vi "Modules - Manual Control.vi"() -> ()   [LabVIEW 2019]
uses:
  Controls/Manual - State.ctl
  Controls/eFGV States.ctl
  Controls/Manual - Data Structure.ctl
  Controls/UDP - Command.ctl
  Controls/Communication - Write Data.ctl
  Controls/Global - IP Address.vi
  Controls/Global - Device.vi
  Controls/Global - Test.vi
  Controls/Global - Channel.vi
  Controls/Global - Unit.vi
  Controls/Global - System.vi
panel:
  in  "Device Name":string
  in  "Zero Ch4":bool
  in  "Zero Ch3":bool
  out "Slide":u8(slide) scale=0.0..1.0
  out "Label Ch4":string caption="Cell Pressure Transducer"
  out "Data Ch4":sgl format="%.2f"
  out "Label Ch3":string caption="Cell Pressure Transducer"
  out "Data Ch3":sgl format="%.2f"
  out "Status":u16(ring) caption="Event" items=["Stop", "Ramp Up", "Ramp Down", "Jog Up", "Jog Down", "PID Mode", "PID Ramp"]
  out "Event":u16(ring) caption="Status" items=["Stop", "Running", "PID", "Up Limit", "Down Limit", "Load Limit"]
  out "Unit Ch2b":string caption="Cell Pressure Transducer"
  in  "Speed":sgl format="%.3f"
  out "Unit Ch2":string caption="Cell Pressure Transducer"
  in  "Setpoint Ch2":sgl
  in  "Target 2":bool
  out "Label Ch1":string caption="Cell Pressure Transducer"
  out "Unit Ch1b":string caption="Cell Pressure Transducer"
  out "Unit Ch1":string caption="Cell Pressure Transducer"
  out "Data Ch2":sgl format="%.3f"
  out "Data Ch1":sgl caption="Load" format="%.3f"
  in  "Setpoint Rate":sgl format="%.3f"
  in  "Stop Ch2":bool
  in  "Ramp":bool
  in  "Zero Ch2":bool
  in  "Setpoint Ch1":sgl
  in  "Stop Ch1":bool
  in  "Target":bool
  in  "Zero Ch1":bool
  in  "Select Machine":u16(ring) items=["Please Select", "TEST"]
  in  "MStop":bool
  in  "Fast down":bool
  in  "Down":bool
  in  "Fast Up":bool
  in  "Up":bool
  out "Label Ch2":string caption="Cell Pressure Transducer"
  # "(         /min)"
  # "/min"
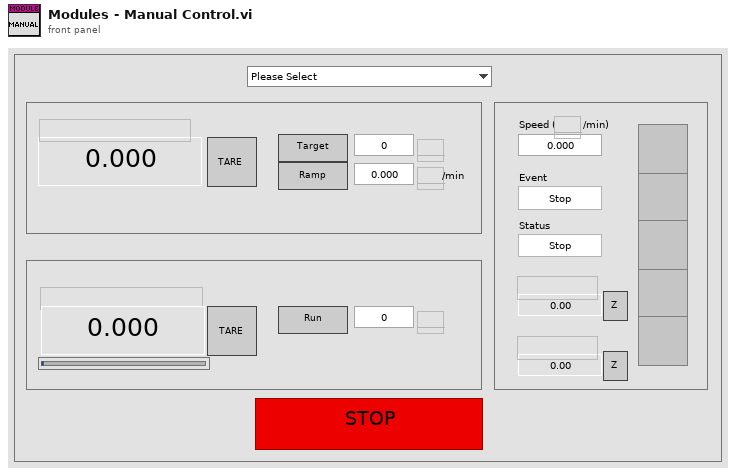
[diagram p1: front panel]
types:
  T1 = enum8{"Enabled", "Disabled", "Disabled and Grayed Out"}
  T2 = typedef "Manual - State.ctl" = enum16{"Init", "Idle", "Read Data", "Stop", "Panel Close", "Close", "Exit"}
  T3 = cluster{"Up":bool, "FUp":bool, "Dn":bool, "FDn":bool, "Running?":bool}
  T4 = typedef "Manual - Data Structure.ctl" = cluster{"Dir":bool, "Device Running?":bool[], "Selected":u16, "PID":cluster{"Output Range":cluster{"High":dbl, "Low":dbl}, "PID Tuning":cluster{"(Kc)":dbl, " (Ti, min)":dbl, "(Td, min)":dbl}, "SetPoint":dbl}, "Machine Table":string[][], "PID Type":enum32{"Sensor", "Displacement"}, "Ramp duration":i32, "i Ramp":i32, "R Elapse":dbl, "R Done":bool, "R To":dbl, "Ramp":bool, "Device Name":string[], "Inv":cluster{"M":i32[], "Bool":bool[]}, "MRun?":bool, "M":cluster{"Up":bool, "FUp":bool, "Dn":bool, "FDn":bool, "Running?":bool}[], "P Target":dbl, "Device IP":string[], "Selected Device":string}
  T5 = enum16{"New Test", "Test Plan", "Job Record", "Instrument", "Machine", "Station", "Machine Control"}
  T6 = typedef "UDP - Command.ctl" = enum16{"Stop", "Jog Up", "Jog Down", "Ramp Up", "Ramp Down", "PID Target", "PID Ramp", "Disp Run", "Read Ch Data", "Zero Channel", "Zero Disp", "Read Sensor", "Write Sensor", "Read ADC", "Write ADC", "Read PID", "Write PID", "Read Test", "Write Test", "Read System", "Write System", "Read Datalog", "Read Datalog Sensor"}
  T7 = typedef "Communication - Write Data.ctl" = cluster{"Test":cluster{"Target Load":sgl, "Target Disp":sgl, "Rate":sgl, "Speed":sgl}, "Sensor":cluster{"Name":string[], "Unit":string[], "Decimal Point":u8[], "Ch Log":u8[], "H Alarm":u8[], "L Alarm":u8[], "H Limit":sgl[], "L Limit":sgl[], "Filter":u8[], "Gain":u8[], "Calib Type":u32[]}, "PID":cluster{"SP":sgl, "PV":sgl, "kP":sgl, "kI":sgl, "kD":sgl, "FF":sgl, "Err Band":sgl, "Max":i32, "Min":i32, "Ts":u32, "Out":i32, "Mode":u8}, "ADC":cluster{"Active Ch":u8[], "Filter Type":u8, "Post Filter":u8[], "Gain":u8[], "FS":u16, "IntOC":u8, "IntFC":u8, "SysOC":u8, "Cofficient":dbl[], "K":dbl[], "Max":i32}, "System":cluster{"Out Type":u8, "Inverse":u8, "Monitor":u8, "Reserve":u8, "ACC Time":u32, "Pulse Rev":u32, "Stroke":u32, "Auto Off":u32, "Gear Ratio":sgl, "Pitch":sgl, "Max Speed":u32, "Jog Speed":u32, "Disp Coff":sgl, "Max Load":u32}, "Index":enum16{"Ch1", "Ch2", "Ch3", "Ch4", "Ch5", "Ch6", "Ch7", "Ch8", "Ch9", "Ch10", "Ch11", "Ch12", "Ch13", "Ch14", "Ch15", "Ch16"}, "Datalog":enum16{"Ch1-Ch16", "Ch17-Ch32", "Ch32-Ch48", "Ch49-Ch64", "Empty"}}
  T8 = enum16{"Ch1", "Ch2", "Ch3", "Ch4", "Ch5", "Ch6", "Ch7", "Ch8", "Ch9", "Ch10", "Ch11", "Ch12", "Ch13", "Ch14", "Ch15", "Ch16"}
  T9 = typedef "eFGV States.ctl" = enum16{"Init", "Read", "Write", "Exit"}
  T10 = cluster{"Up":bool, "FUp":bool, "Dn":bool, "FDn":bool, "Running?":bool}[]
  T11 = cluster{"Target Load":sgl, "Target Disp":sgl, "Rate":sgl, "Speed":sgl}[]
  T12 = cluster{"Target Load":sgl, "Target Disp":sgl, "Rate":sgl, "Speed":sgl}
  T13 = cluster{"Out Type":u8, "Inverse":u8, "Monitor":u8, "Reserve":u8, "ACC Time":u32, "Pulse Rev":u32, "Stroke":u32, "Auto Off":u32, "Gear Ratio":sgl, "Pitch":sgl, "Max Speed":u32, "Jog Speed":u32, "Disp Coff":sgl, "Max Load":u32}[]
  T14 = typedef "UDP - Event.ctl" = u16
  T15 = typedef "UDP - Status.ctl" = u16
  T16 = cluster{"Channels":cluster{"Ch1":sgl, "Ch2":sgl, "Ch3":sgl, "Ch4":sgl, "Ch5":sgl, "Ch6":sgl, "Ch7":sgl, "Ch8":sgl, "Ch9":sgl, "Ch10":sgl, "Ch11":sgl, "Ch12":sgl, "Ch13":sgl, "Ch14":sgl, "Ch15":sgl, "Ch16":sgl}, "Event":T14, "Status":T15, "IP":string}[]
  T17 = cluster{"Channels":cluster{"Ch1":sgl, "Ch2":sgl, "Ch3":sgl, "Ch4":sgl, "Ch5":sgl, "Ch6":sgl, "Ch7":sgl, "Ch8":sgl, "Ch9":sgl, "Ch10":sgl, "Ch11":sgl, "Ch12":sgl, "Ch13":sgl, "Ch14":sgl, "Ch15":sgl, "Ch16":sgl}, "Event":T14, "Status":T15, "IP":string}
  T18 = cluster{"Out Type":u8, "Inverse":u8, "Monitor":u8, "Reserve":u8, "ACC Time":u32, "Pulse Rev":u32, "Stroke":u32, "Auto Off":u32, "Gear Ratio":sgl, "Pitch":sgl, "Max Speed":u32, "Jog Speed":u32, "Disp Coff":sgl, "Max Load":u32}
  T19 = cluster{"Name":string[], "Unit":string[], "Decimal Point":u8[], "Ch Log":u8[], "H Alarm":u8[], "L Alarm":u8[], "H Limit":sgl[], "L Limit":sgl[], "Filter":u8[], "Gain":u8[], "Calib Type":u32[]}[]
  T20 = cluster{"Name":string[], "Unit":string[], "Decimal Point":u8[], "Ch Log":u8[], "H Alarm":u8[], "L Alarm":u8[], "H Limit":sgl[], "L Limit":sgl[], "Filter":u8[], "Gain":u8[], "Calib Type":u32[]}
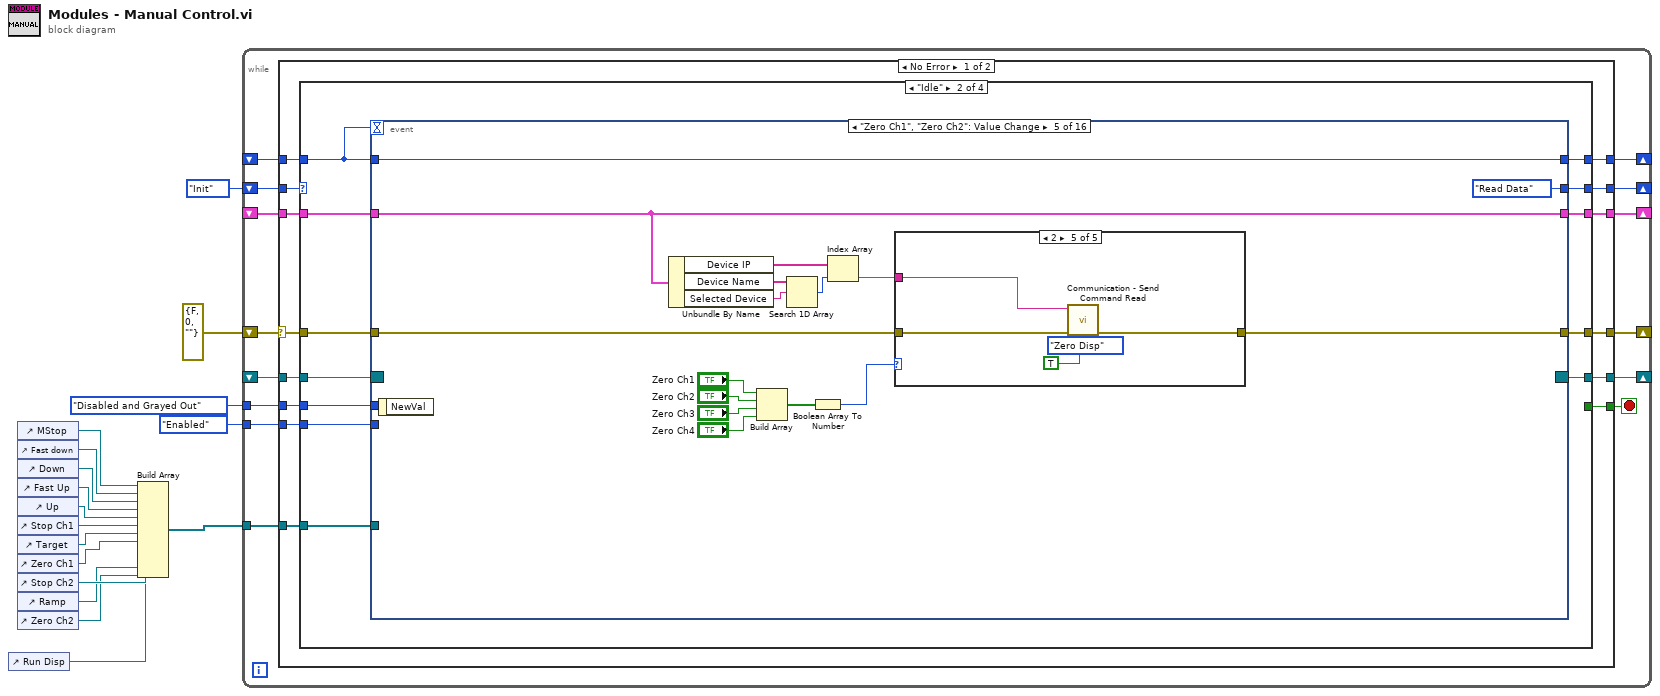
[diagram p0: block diagram]
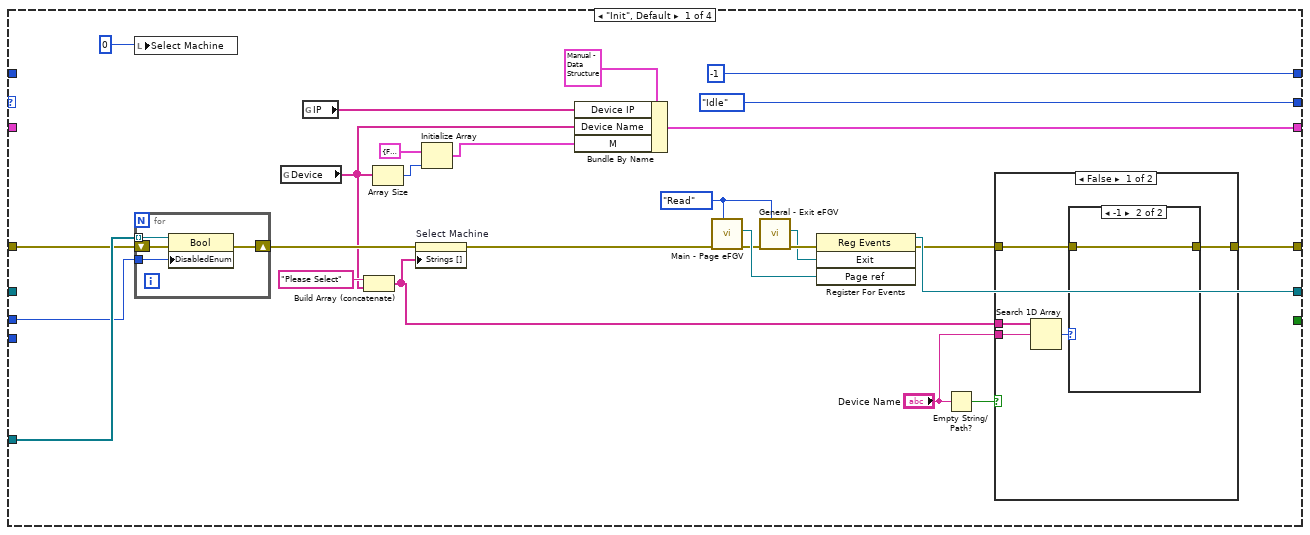
[diagram p2: hidden frame]
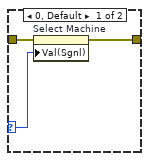
[diagram p3: hidden frame]
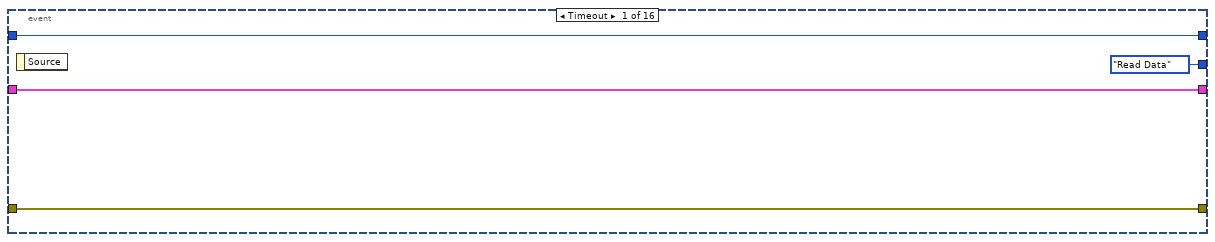
[diagram p5: hidden frame]
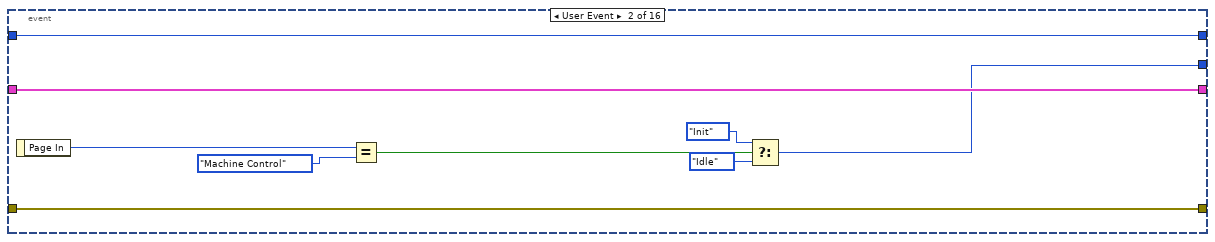
[diagram p6: hidden frame]
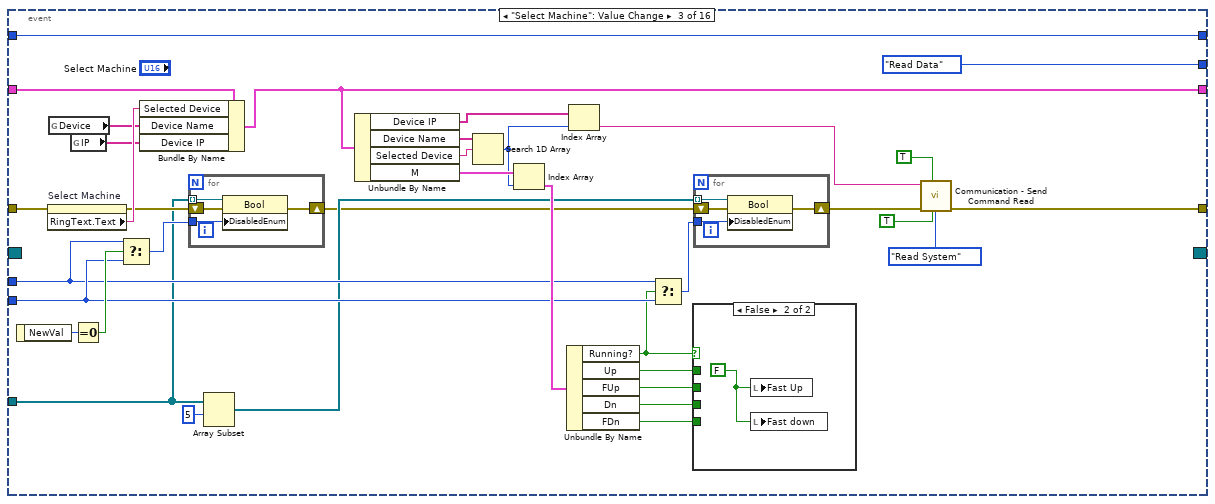
[diagram p7: hidden frame]
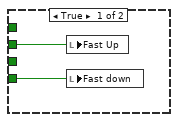
[diagram p8: hidden frame]
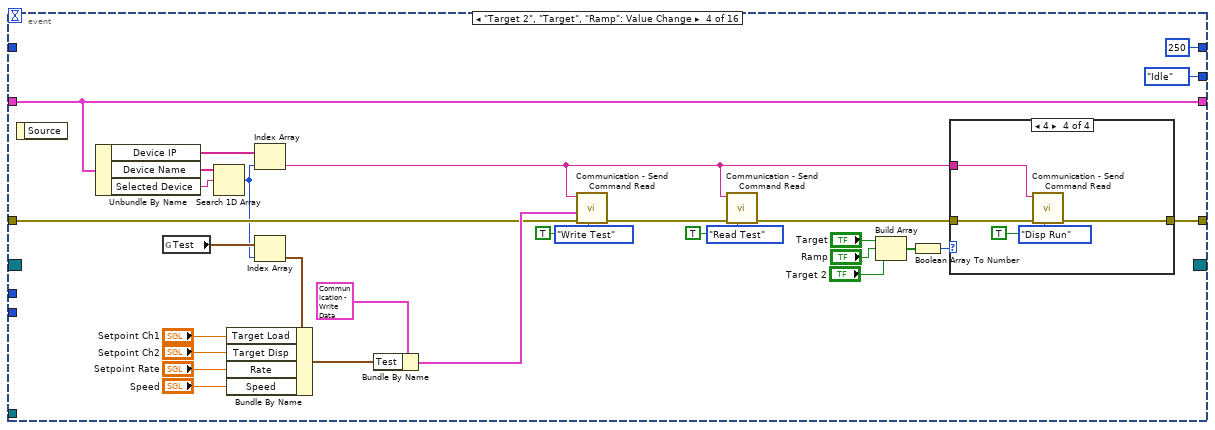
[diagram p9: hidden frame]
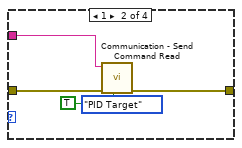
[diagram p11: hidden frame]
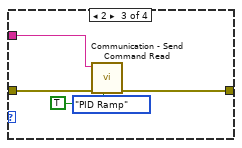
[diagram p12: hidden frame]
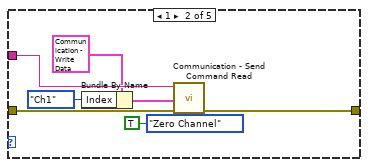
[diagram p14: hidden frame]
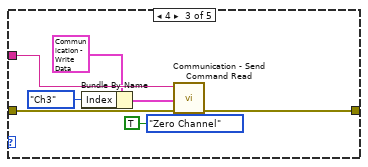
[diagram p15: hidden frame]
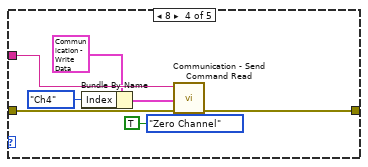
[diagram p16: hidden frame]
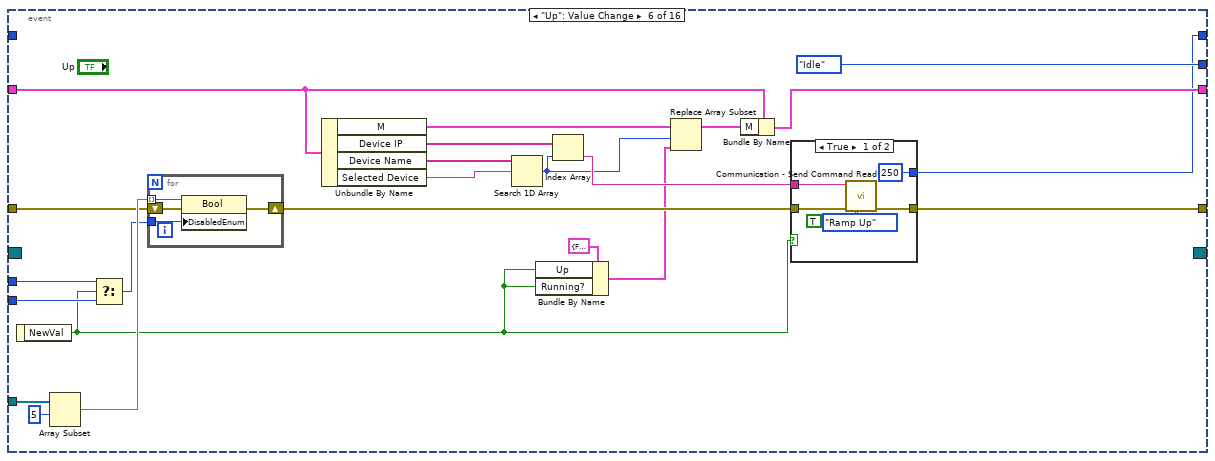
[diagram p17: hidden frame]
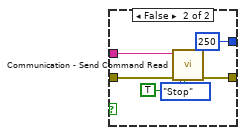
[diagram p18: hidden frame]
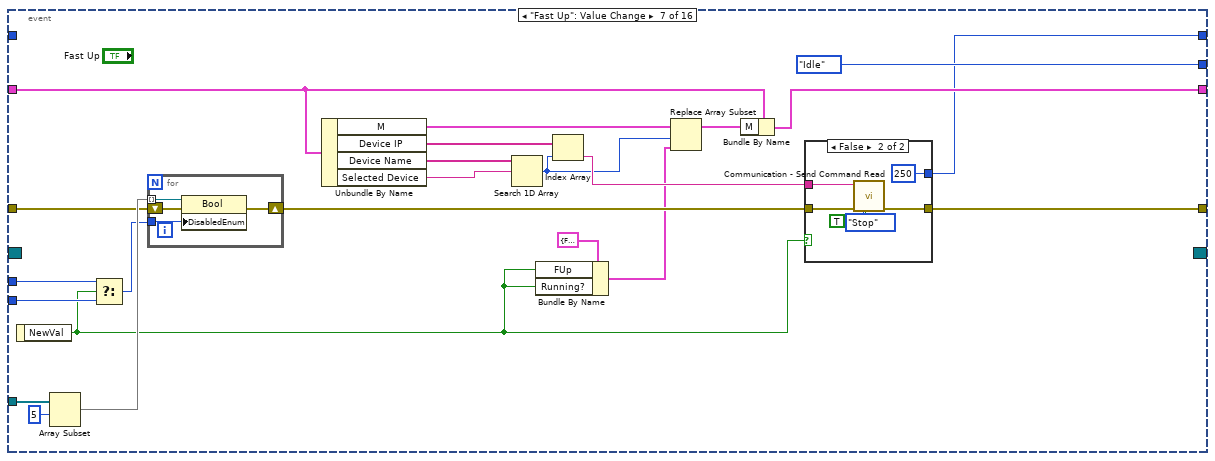
[diagram p19: hidden frame]
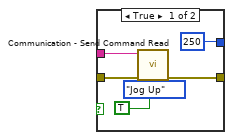
[diagram p20: hidden frame]
diagram:
  n1 = control-ref of="Run Disp"() -> (w1:refnum<vi>)
  n2 = control-ref of="MStop"() -> (w15:refnum<vi>)
  n3 = control-ref of="Fast down"() -> (w14:refnum<vi>)
  n4 = control-ref of="Down"() -> (w13:refnum<vi>)
  n5 = control-ref of="Fast Up"() -> (w12:refnum<vi>)
  n6 = control-ref of="Up"() -> (w11:refnum<vi>)
  n7 = control-ref of="Stop Ch1"() -> (w10:refnum<vi>)
  n8 = control-ref of="Target"() -> (w9:refnum<vi>)
  n9 = control-ref of="Zero Ch1"() -> (w8:refnum<vi>)
  n10 = control-ref of="Stop Ch2"() -> (w7:refnum<vi>)
  n11 = control-ref of="Ramp"() -> (w6:refnum<vi>)
  n12 = control-ref of="Zero Ch2"() -> (w5:refnum<vi>)
  n13 = Build Array(w15, w14, w13, w12, w11, w10, w9, w8, w7, w6, w5, w1) -> (w4:refnum<vi>[])
  n14 = while {
    shift-right: [w29] -> _
    shift-left: errorcluster {"status"=FALSE, "code"=0, "source"=""} ("error constant") -> [w31]
    shift-right: [w28] -> _
    shift-left: Manual_-_State."Init" -> [w30]
    shift-right: [w26] -> _
    shift-left: _ -> [w25]
    shift-right: [w24] -> _
    shift-left: _ -> [w23]
    shift-right: [w22] -> _
    shift-left: _ -> [w21]
    tunnel: w4 -> [w20]
    tunnel: T1."Disabled and Grayed Out" ("Disabled") -> [w19]
    tunnel: T1."Enabled" ("Disabled") -> [w18]
    stop <- w27 stop-if-true
    n15 = case shown="No Error" w31 {
      selector: w31 -> [w43 w617]
      tunnel: w30 -> [w45 _]
      tunnel: [w44 w618] -> w29
      tunnel: [w42 Manual_-_State."Idle"] -> w28
      tunnel: [w41 _] -> w27
      tunnel: [w40 w625] -> w26
      tunnel: w25 -> [w39 w625]
      tunnel: [w38 w628] -> w24
      tunnel: w23 -> [w37 w628]
      tunnel: [w36 w627] -> w22
      tunnel: w21 -> [w35 w627]
      tunnel: w20 -> [w34 _]
      tunnel: w19 -> [w33 _]
      tunnel: w18 -> [w32 _]
      frame No Error {
        n16 = case shown="\"Idle\"" w45 {
          tunnel: [w49 w92 w577 w610] -> w44
          tunnel: w43 -> [w51 w91 w566 w609]
          tunnel: [Manual_-_State."Idle" w98 Manual_-_State."Idle" Manual_-_State."Close"] -> w42
          tunnel: [_ _ _ TRUE] -> w41
          tunnel: [-1 w97 w596 -1] -> w40
          tunnel: w39 -> [_ w87 w596 _]
          tunnel: [w68 w95 w595 w613] -> w38
          tunnel: w37 -> [_ w96 w595 w613]
          tunnel: [w57 w94 w593 T4 {"Dir"=FALSE, "Device Running?"=[], "Selected"=0, "PID"={"Output Range"={"High"=100.0, "Low"=-100.0}, "PID Tuning"={"(Kc)"=1.0, " (Ti, min)"=0.01, "(Td, min)"=0.0}, "SetPoint"=0.0}, "Machine Table"=[], "PID Type"=enum."Sensor", "Ramp duration"=0, "i Ramp"=0, "R Elapse"=0.0, "R Done"=FALSE, "R To"=0.0, "Ramp"=FALSE, "Device Name"=[], "Inv"={"M"=[], "Bool"=[]}, "MRun?"=FALSE, "M"=[], "P Target"=0.0, "Device IP"=[], "Selected Device"=""}] -> w36
          tunnel: w35 -> [_ w93 w593 _]
          tunnel: w34 -> [w64 w90 _ _]
          tunnel: w33 -> [w62 w89 _ _]
          tunnel: w32 -> [_ w88 _ _]
          frame "Init", Default {
            w65 = eFGV_States."Read" ("Action")
            n17 = local write "Select Machine"(0) -> ()
            n18 = for {
              shift-right: [w85] -> w60
              shift-left: w51 -> [w86]
              tunnel: w64 -> [w84] mode=indexing
              tunnel: w62 -> [w83]
              n19 = property class="Bool"(reference=w84, error in=w86, "DisabledEnum"=w83) -> (error out=w85:errorcluster)  [unwired: 1 out]
            }
            n20 = global read "Global - Device.vi" "Device"() -> (w53:string[])
            n21 = global read "Global - IP Address.vi" "IP"() -> (w52:string[])
            n22 = Build Array (concatenate)("Please Select", w53) -> (w47:string[])
            n23 = Array Size(array=w53) -> (size(s)=w56:i32)
            n24 = property on="Select Machine" class="Ring (strict)"(error in=w60, "Strings []"=w47) -> (error out=w59:errorcluster)  [unwired: 1 in, 1 out]
            n25 = Initialize Array(T3 {"Up"=FALSE, "FUp"=FALSE, "Dn"=FALSE, "FDn"=FALSE, "Running?"=FALSE} ("M"), w56) -> (w54:T10)
            n26 = Bundle By Name(cluster=T4 {"Dir"=FALSE, "Device Running?"=[], "Selected"=0, "PID"={"Output Range"={"High"=100.0, "Low"=-100.0}, "PID Tuning"={"(Kc)"=1.0, " (Ti, min)"=0.01, "(Td, min)"=0.0}, "SetPoint"=0.0}, "Machine Table"=[], "PID Type"=enum."Sensor", "Ramp duration"=0, "i Ramp"=0, "R Elapse"=0.0, "R Done"=FALSE, "R To"=0.0, "Ramp"=FALSE, "Device Name"=[], "Inv"={"M"=[], "Bool"=[]}, "MRun?"=FALSE, "M"=[], "P Target"=0.0, "Device IP"=[], "Selected Device"=""}, "Device IP"=w52, "Device Name"=w53, "M"=w54) -> (w57:T4)
            n27 = call "Main - Page eFGV.vi"("eFGV States"=w65, "error in (no error)"=w59) -> ("error out"=w63:errorcluster, "Page ref"=w66:refnum<user-event>)  [unwired: 7 in, 1 out]
            n28 = call "General - Exit eFGV.vi"("eFGV States"=w65, "error in (no error)"=w63) -> ("error out"=w70:errorcluster, "Exit"=w69:refnum<user-event>)  [unwired: 7 in, 1 out]
            n29 = register-events(error in=w70, w69, w66) -> (reference out=w68:refnum<event-registration>, error out=w48:errorcluster)  [unwired: 1 in]
            n30 = Empty String/Path?(string/path="Device Name") -> (empty?=w50:bool)
            n31 = case shown="False" w50 {
              tunnel: [w74 w82] -> w49
              tunnel: w48 -> [w75 w82]
              tunnel: w47 -> [w77 _]
              tunnel: "Device Name" -> [w76 _]
              frame False {
                n32 = Search 1D Array(1D array=w77, element=w76) -> (index of element=w73:i32)  [unwired: 1 in]
                n33 = case shown="-1" w73 {
                  selector: w73 -> [w78 _]
                  tunnel: w75 -> [w80 w81]
                  tunnel: [w79 w81] -> w74
                  frame 0, Default {
                    n34 = property on="Select Machine" class="Ring (strict)"(error in=w80, "Val(Sgnl)"=w78) -> (error out=w79:errorcluster)  [unwired: 1 in, 1 out]
                  }
                  frame -1 {
                  }
                }
              }
              frame True {
              }
            }
          }
          frame "Idle" {
            n35 = event shown="[4] \"Zero Ch1\", \"Zero Ch2\": Value Change" {
              selector: w96 -> [_ _ _ _ _ _ _ _ _ _ _ _ _ _ _ _]
              dyn-events: [_ _ _ _ _ _ _ _ _ _ _ _ _ _ _ _] -> w95
              timeout: w87 -> [_ _ _ _ _ _ _ _ _ _ _ _ _ _ _ _]
              tunnel: [w102 w111 w116 w183 w207 w252 w300 w339 w378 w423 w434 w455 w476 w497 w521 w537] -> w92
              tunnel: w91 -> [w102 w111 w144 w165 w211 w267 w306 w345 w384 w428 w450 w471 w492 w513 w520 w538]
              tunnel: [Manual_-_State."Read Data" w104 Manual_-_State."Read Data" Manual_-_State."Idle" Manual_-_State."Read Data" Manual_-_State."Idle" Manual_-_State."Idle" Manual_-_State."Idle" Manual_-_State."Idle" Manual_-_State."Idle" Manual_-_State."Idle" Manual_-_State."Idle" Manual_-_State."Idle" Manual_-_State."Idle" Manual_-_State."Close" Manual_-_State."Idle"] -> w98
              tunnel: [w99 w103 w124 250 ("f") w220 w251 w290 w329 w368 250 ("f") w454 w475 w496 w517 -1 w530] -> w97
              tunnel: w87 -> [w99 w103 w124 _ w220 _ _ _ _ _ w454 w475 w496 w517 _ w529]
              tunnel: [w100 w110 w139 w179 w210 w261 w299 w338 w377 w422 w446 w467 w488 w509 w519 w539] -> w94
              tunnel: w93 -> [w100 w110 w146 w179 w210 w260 w298 w337 w376 w421 w446 w467 w488 w509 w519 w539]
              tunnel: w90 -> [_ _ w132 _ _ w270 w309 w348 w387 w414 _ _ _ _ _ _]
              tunnel: w89 -> [_ _ w134 _ _ w269 w308 w347 w386 _ _ _ _ _ _ _]
              tunnel: w88 -> [_ _ w135 _ _ w268 w307 w346 w385 w415 _ _ _ _ _ _]
              event Timeout {
                n36 = event-data() -> ()  [unwired: 1 in, 1 out]
              }
              event User Event {
                n37 = event-data() -> ("Page In"=w108:T5)  [unwired: 1 in]
                n38 = Equal?(x=w108, y=T5."Machine Control" ("Page In")) -> (x = y?=w107:bool)
                n39 = Select(t=Manual_-_State."Init", s=w107, f=Manual_-_State."Idle") -> (s? t:f=w104:T2)
              }
              event "Select Machine": Value Change {
                n40 = event-data() -> ("NewVal"=w141:u16)  [unwired: 1 in]
                n41 = property on="Select Machine" class="Ring (strict)"(error in=w144) -> (error out=w138:errorcluster, "RingText.Text"=w145:string)  [unwired: 1 in, 1 out]
                n42 = global read "Global - Device.vi" "Device"() -> (w122:string[])
                n43 = global read "Global - IP Address.vi" "IP"() -> (w121:string[])
                n44 = Equal To 0?(x=w141) -> (x = 0?=w143:bool)
                n45 = Select(t=w134, s=w143, f=w135) -> (s? t:f=w142:T1)
                n46 = Bundle By Name(cluster=w146, "Selected Device"=w145, "Device Name"=w122, "Device IP"=w121) -> (w139:T4)
                n47 = for {
                  shift-right: [w157] -> w123
                  shift-left: w138 -> [w158]
                  tunnel: w132 -> [w156] mode=indexing
                  tunnel: w142 -> [w155]
                  n48 = property class="Bool"(reference=w156, error in=w158, "DisabledEnum"=w155) -> (error out=w157:errorcluster)  [unwired: 1 out]
                }
                n49 = Array Subset(array=w132, index=5) -> (w130:refnum<vi>[])  [unwired: 1 in]
                n50 = Unbundle By Name(w139) -> ("Device IP"=w114:string[], "Device Name"=w120:string[], "Selected Device"=w140:string, "M"=w137:T10)
                n51 = Search 1D Array(1D array=w120, element=w140) -> (index of element=w113:i32)  [unwired: 1 in]
                n52 = Index Array(array=w137, index=w113) -> (element=w136:T3)
                n53 = Unbundle By Name(w136) -> ("Running?"=w125:bool, "Up"=w129:bool, "FUp"=w128:bool, "Dn"=w127:bool, "FDn"=w126:bool)
                n54 = Index Array(array=w114, index=w113) -> (element=w112:string)
                n55 = Select(t=w134, s=w125, f=w135) -> (s? t:f=w131:T1)
                n56 = case shown="False" w125 {
                  tunnel: w129 -> [_ _]
                  tunnel: w128 -> [w149 _]
                  tunnel: w127 -> [_ _]
                  tunnel: w126 -> [w148 _]
                  frame True {
                    n57 = local write "Fast Up"(w149) -> ()
                    n58 = local write "Fast down"(w148) -> ()
                  }
                  frame False {
                    w150 = FALSE ("Up")
                    n59 = local write "Fast Up"(w150) -> ()
                    n60 = local write "Fast down"(w150) -> ()
                  }
                }
                n61 = for {
                  shift-right: [w153] -> w117
                  shift-left: w123 -> [w154]
                  tunnel: w130 -> [w152] mode=indexing
                  tunnel: w131 -> [w151]
                  n62 = property class="Bool"(reference=w152, error in=w154, "DisabledEnum"=w151) -> (error out=w153:errorcluster)  [unwired: 1 out]
                }
                n63 = call "Communication - Send Command Read.vi"("Fron?"=TRUE, "Bypass?"=TRUE, "error in (no error)"=w117, "Action"=UDP_-_Command."Read System", "Device IP Address"=w112) -> ("error out"=w116:errorcluster)  [unwired: 6 in]
              }
              event "Target 2", "Target", "Ramp": Value Change {
                n64 = event-data() -> ()  [unwired: 1 in, 1 out]
                n65 = Unbundle By Name(w179) -> ("Device IP"=w180:string[], "Device Name"=w182:string[], "Selected Device"=w181:string)
                n66 = global read "Global - Test.vi" "Test"() -> (w173:T11)
                n67 = Search 1D Array(1D array=w182, element=w181) -> (index of element=w163:i32)  [unwired: 1 in]
                n68 = Index Array(array=w180, index=w163) -> (element=w164:string)
                n69 = Index Array(array=w173, index=w163) -> (element=w172:T12)
                n70 = Bundle By Name(cluster=w172, "Target Load"="Setpoint Ch1", "Target Disp"="Setpoint Ch2", "Rate"="Setpoint Rate", "Speed"="Speed") -> (w171:T12)
                n71 = Bundle By Name(cluster=T7 {"Test"={"Target Load"=0.0, "Target Disp"=0.0, "Rate"=0.0, "Speed"=0.0}, "Sensor"={"Name"=[], "Unit"=[], "Decimal Point"=[], "Ch Log"=[], "H Alarm"=[], "L Alarm"=[], "H Limit"=[], "L Limit"=[], "Filter"=[], "Gain"=[], "Calib Type"=[]}, "PID"={"SP"=0.0, "PV"=0.0, "kP"=0.0, "kI"=0.0, "kD"=0.0, "FF"=0.0, "Err Band"=0.0, "Max"=0, "Min"=0, "Ts"=0, "Out"=0, "Mode"=0}, "ADC"={"Active Ch"=[], "Filter Type"=0, "Post Filter"=[], "Gain"=[], "FS"=0, "IntOC"=0, "IntFC"=0, "SysOC"=0, "Cofficient"=[], "K"=[], "Max"=0}, "System"={"Out Type"=0, "Inverse"=0, "Monitor"=0, "Reserve"=0, "ACC Time"=0, "Pulse Rev"=0, "Stroke"=0, "Auto Off"=0, "Gear Ratio"=0.0, "Pitch"=0.0, "Max Speed"=0, "Jog Speed"=0, "Disp Coff"=0.0, "Max Load"=0}, "Index"=enum."Ch1", "Datalog"=enum."Ch1-Ch16"} ("Data"), "Test"=w171) -> (w170:T7)
                n72 = call "Communication - Send Command Read.vi"("Fron?"=TRUE, "error in (no error)"=w165, "Data"=w170, "Action"=UDP_-_Command."Write Test", "Device IP Address"=w164) -> ("error out"=w167:errorcluster)  [unwired: 6 in]
                n73 = call "Communication - Send Command Read.vi"("Fron?"=TRUE, "error in (no error)"=w167, "Action"=UDP_-_Command."Read Test", "Device IP Address"=w164) -> ("error out"=w166:errorcluster)  [unwired: 7 in]
                n74 = Build Array("Target", "Ramp", "Target 2") -> (w186:bool[])
                n75 = Boolean Array To Number(Boolean array=w186) -> (number=w184:u32)
                n76 = case shown="4" w184 {
                  tunnel: w166 -> [w189 w190 w196 w201]
                  tunnel: [w189 w193 w198 w203] -> w183
                  tunnel: w164 -> [_ w192 w197 w202]
                  frame Default {
                  }
                  frame 1 {
                    n77 = call "Communication - Send Command Read.vi"("Fron?"=TRUE, "error in (no error)"=w190, "Action"=UDP_-_Command."PID Target", "Device IP Address"=w192) -> ("error out"=w193:errorcluster)  [unwired: 7 in]
                  }
                  frame 2 {
                    n78 = call "Communication - Send Command Read.vi"("Fron?"=TRUE, "error in (no error)"=w196, "Action"=UDP_-_Command."PID Ramp", "Device IP Address"=w197) -> ("error out"=w198:errorcluster)  [unwired: 7 in]
                  }
                  frame 4 {
                    n79 = call "Communication - Send Command Read.vi"("Fron?"=TRUE, "error in (no error)"=w201, "Action"=UDP_-_Command."Disp Run", "Device IP Address"=w202) -> ("error out"=w203:errorcluster)  [unwired: 7 in]
                  }
                }
              }
              event "Zero Ch1", "Zero Ch2": Value Change {
                n80 = event-data() -> ()  [unwired: 1 in, 1 out]
                n81 = Unbundle By Name(w210) -> ("Device IP"=w213:string[], "Device Name"=w215:string[], "Selected Device"=w214:string)
                n82 = Build Array("Zero Ch1", "Zero Ch2", "Zero Ch3", "Zero Ch4") -> (w219:bool[])
                n83 = Search 1D Array(1D array=w215, element=w214) -> (index of element=w212:i32)  [unwired: 1 in]
                n84 = Boolean Array To Number(Boolean array=w219) -> (number=w209:u32)
                n85 = Index Array(array=w213, index=w212) -> (element=w208:string)
                n86 = case shown="2" w209 {
                  tunnel: w211 -> [w221 w229 w237 w245 w250]
                  tunnel: [w221 w228 w236 w244 w246] -> w207
                  tunnel: w208 -> [_ w227 w235 w243 w249]
                  frame Default {
                  }
                  frame 1 {
                    n87 = Bundle By Name(cluster=T7 {"Test"={"Target Load"=0.0, "Target Disp"=0.0, "Rate"=0.0, "Speed"=0.0}, "Sensor"={"Name"=[], "Unit"=[], "Decimal Point"=[], "Ch Log"=[], "H Alarm"=[], "L Alarm"=[], "H Limit"=[], "L Limit"=[], "Filter"=[], "Gain"=[], "Calib Type"=[]}, "PID"={"SP"=0.0, "PV"=0.0, "kP"=0.0, "kI"=0.0, "kD"=0.0, "FF"=0.0, "Err Band"=0.0, "Max"=0, "Min"=0, "Ts"=0, "Out"=0, "Mode"=0}, "ADC"={"Active Ch"=[], "Filter Type"=0, "Post Filter"=[], "Gain"=[], "FS"=0, "IntOC"=0, "IntFC"=0, "SysOC"=0, "Cofficient"=[], "K"=[], "Max"=0}, "System"={"Out Type"=0, "Inverse"=0, "Monitor"=0, "Reserve"=0, "ACC Time"=0, "Pulse Rev"=0, "Stroke"=0, "Auto Off"=0, "Gear Ratio"=0.0, "Pitch"=0.0, "Max Speed"=0, "Jog Speed"=0, "Disp Coff"=0.0, "Max Load"=0}, "Index"=enum."Ch1", "Datalog"=enum."Ch1-Ch16"} ("Data"), "Index"=T8."Ch1" ("Zero")) -> (w223:T7)
                    n88 = call "Communication - Send Command Read.vi"("Fron?"=TRUE, "error in (no error)"=w229, "Data"=w223, "Action"=UDP_-_Command."Zero Channel", "Device IP Address"=w227) -> ("error out"=w228:errorcluster)  [unwired: 6 in]
                  }
                  frame 4 {
                    n89 = Bundle By Name(cluster=T7 {"Test"={"Target Load"=0.0, "Target Disp"=0.0, "Rate"=0.0, "Speed"=0.0}, "Sensor"={"Name"=[], "Unit"=[], "Decimal Point"=[], "Ch Log"=[], "H Alarm"=[], "L Alarm"=[], "H Limit"=[], "L Limit"=[], "Filter"=[], "Gain"=[], "Calib Type"=[]}, "PID"={"SP"=0.0, "PV"=0.0, "kP"=0.0, "kI"=0.0, "kD"=0.0, "FF"=0.0, "Err Band"=0.0, "Max"=0, "Min"=0, "Ts"=0, "Out"=0, "Mode"=0}, "ADC"={"Active Ch"=[], "Filter Type"=0, "Post Filter"=[], "Gain"=[], "FS"=0, "IntOC"=0, "IntFC"=0, "SysOC"=0, "Cofficient"=[], "K"=[], "Max"=0}, "System"={"Out Type"=0, "Inverse"=0, "Monitor"=0, "Reserve"=0, "ACC Time"=0, "Pulse Rev"=0, "Stroke"=0, "Auto Off"=0, "Gear Ratio"=0.0, "Pitch"=0.0, "Max Speed"=0, "Jog Speed"=0, "Disp Coff"=0.0, "Max Load"=0}, "Index"=enum."Ch1", "Datalog"=enum."Ch1-Ch16"} ("Data"), "Index"=T8."Ch3" ("Zero")) -> (w231:T7)
                    n90 = call "Communication - Send Command Read.vi"("Fron?"=TRUE, "error in (no error)"=w237, "Data"=w231, "Action"=UDP_-_Command."Zero Channel", "Device IP Address"=w235) -> ("error out"=w236:errorcluster)  [unwired: 6 in]
                  }
                  frame 8 {
                    n91 = Bundle By Name(cluster=T7 {"Test"={"Target Load"=0.0, "Target Disp"=0.0, "Rate"=0.0, "Speed"=0.0}, "Sensor"={"Name"=[], "Unit"=[], "Decimal Point"=[], "Ch Log"=[], "H Alarm"=[], "L Alarm"=[], "H Limit"=[], "L Limit"=[], "Filter"=[], "Gain"=[], "Calib Type"=[]}, "PID"={"SP"=0.0, "PV"=0.0, "kP"=0.0, "kI"=0.0, "kD"=0.0, "FF"=0.0, "Err Band"=0.0, "Max"=0, "Min"=0, "Ts"=0, "Out"=0, "Mode"=0}, "ADC"={"Active Ch"=[], "Filter Type"=0, "Post Filter"=[], "Gain"=[], "FS"=0, "IntOC"=0, "IntFC"=0, "SysOC"=0, "Cofficient"=[], "K"=[], "Max"=0}, "System"={"Out Type"=0, "Inverse"=0, "Monitor"=0, "Reserve"=0, "ACC Time"=0, "Pulse Rev"=0, "Stroke"=0, "Auto Off"=0, "Gear Ratio"=0.0, "Pitch"=0.0, "Max Speed"=0, "Jog Speed"=0, "Disp Coff"=0.0, "Max Load"=0}, "Index"=enum."Ch1", "Datalog"=enum."Ch1-Ch16"} ("Data"), "Index"=T8."Ch4" ("Zero")) -> (w239:T7)
                    n92 = call "Communication - Send Command Read.vi"("Fron?"=TRUE, "error in (no error)"=w245, "Data"=w239, "Action"=UDP_-_Command."Zero Channel", "Device IP Address"=w243) -> ("error out"=w244:errorcluster)  [unwired: 6 in]
                  }
                  frame 2 {
                    n93 = call "Communication - Send Command Read.vi"("Fron?"=TRUE, "error in (no error)"=w250, "Action"=UDP_-_Command."Zero Disp", "Device IP Address"=w249) -> ("error out"=w246:errorcluster)  [unwired: 7 in]
                  }
                }
              }
              event "Up": Value Change {
                n94 = event-data() -> ("NewVal"=w257:bool)  [unwired: 1 in]
                n95 = Array Subset(array=w270, index=5) -> (w272:refnum<vi>[])  [unwired: 1 in]
                n96 = Select(t=w269, s=w257, f=w268) -> (s? t:f=w266:T1)
                n97 = for {
                  shift-right: [w288] -> w265
                  shift-left: w267 -> [w289]
                  tunnel: w272 -> [w287] mode=indexing
                  tunnel: w266 -> [w286]
                  n98 = property class="Bool"(reference=w287, error in=w289, "DisabledEnum"=w286) -> (error out=w288:errorcluster)  [unwired: 1 out]
                }
                n99 = Unbundle By Name(w260) -> ("M"=w258:T10, "Device IP"=w263:string[], "Device Name"=w264:string[], "Selected Device"=w256:string)
                n100 = Search 1D Array(1D array=w264, element=w256) -> (index of element=w254:i32)  [unwired: 1 in]
                n101 = Bundle By Name(cluster=T3 {"Up"=FALSE, "FUp"=FALSE, "Dn"=FALSE, "FDn"=FALSE, "Running?"=FALSE} ("element"), "Up"=w257, "Running?"=w257) -> (w255:T3)
                n102 = Index Array(array=w263, index=w254) -> (element=w262:string)
                n103 = Replace Array Subset(array=w258, new element=w255, index=w254) -> (w259:T10)
                n104 = Bundle By Name(cluster=w260, "M"=w259) -> (w261:T4)
                n105 = case shown="True" w257 {
                  tunnel: w265 -> [w279 w285]
                  tunnel: [w277 w284] -> w252
                  tunnel: w262 -> [w278 w283]
                  tunnel: [250 ("f") 250 ("f")] -> w251
                  frame True {
                    n106 = call "Communication - Send Command Read.vi"("Fron?"=TRUE, "error in (no error)"=w279, "Action"=UDP_-_Command."Ramp Up", "Device IP Address"=w278) -> ("error out"=w277:errorcluster)  [unwired: 7 in]
                  }
                  frame False {
                    n107 = call "Communication - Send Command Read.vi"("Fron?"=TRUE, "error in (no error)"=w285, "Action"=UDP_-_Command."Stop", "Device IP Address"=w283) -> ("error out"=w284:errorcluster)  [unwired: 7 in]
                  }
                }
              }
              event "Fast Up": Value Change {
                n108 = event-data() -> ("NewVal"=w295:bool)  [unwired: 1 in]
                n109 = Array Subset(array=w309, index=5) -> (w311:refnum<vi>[])  [unwired: 1 in]
                n110 = Select(t=w308, s=w295, f=w307) -> (s? t:f=w305:T1)
                n111 = for {
                  shift-right: [w327] -> w304
                  shift-left: w306 -> [w328]
                  tunnel: w311 -> [w326] mode=indexing
                  tunnel: w305 -> [w325]
                  n112 = property class="Bool"(reference=w326, error in=w328, "DisabledEnum"=w325) -> (error out=w327:errorcluster)  [unwired: 1 out]
                }
                n113 = Unbundle By Name(w298) -> ("M"=w296:T10, "Device IP"=w302:string[], "Device Name"=w303:string[], "Selected Device"=w294:string)
                n114 = Search 1D Array(1D array=w303, element=w294) -> (index of element=w292:i32)  [unwired: 1 in]
                n115 = Bundle By Name(cluster=T3 {"Up"=FALSE, "FUp"=FALSE, "Dn"=FALSE, "FDn"=FALSE, "Running?"=FALSE} ("element"), "FUp"=w295, "Running?"=w295) -> (w293:T3)
                n116 = Index Array(array=w302, index=w292) -> (element=w301:string)
                n117 = Replace Array Subset(array=w296, new element=w293, index=w292) -> (w297:T10)
                n118 = Bundle By Name(cluster=w298, "M"=w297) -> (w299:T4)
                n119 = case shown="False" w295 {
                  tunnel: w304 -> [w318 w324]
                  tunnel: [w317 w323] -> w300
                  tunnel: w301 -> [w316 w322]
                  tunnel: [250 ("f") 250 ("f")] -> w290
                  frame True {
                    n120 = call "Communication - Send Command Read.vi"("Fron?"=TRUE, "error in (no error)"=w318, "Action"=UDP_-_Command."Jog Up", "Device IP Address"=w316) -> ("error out"=w317:errorcluster)  [unwired: 7 in]
                  }
                  frame False {
                    n121 = call "Communication - Send Command Read.vi"("Fron?"=TRUE, "error in (no error)"=w324, "Action"=UDP_-_Command."Stop", "Device IP Address"=w322) -> ("error out"=w323:errorcluster)  [unwired: 7 in]
                  }
                }
              }
              event "Down": Value Change {
                n122 = event-data() -> ("NewVal"=w334:bool)  [unwired: 1 in]
                n123 = Array Subset(array=w348, index=5) -> (w350:refnum<vi>[])  [unwired: 1 in]
                n124 = Select(t=w347, s=w334, f=w346) -> (s? t:f=w344:T1)
                n125 = for {
                  shift-right: [w366] -> w343
                  shift-left: w345 -> [w367]
                  tunnel: w350 -> [w365] mode=indexing
                  tunnel: w344 -> [w364]
                  n126 = property class="Bool"(reference=w365, error in=w367, "DisabledEnum"=w364) -> (error out=w366:errorcluster)  [unwired: 1 out]
                }
                n127 = Unbundle By Name(w337) -> ("M"=w335:T10, "Device IP"=w341:string[], "Device Name"=w342:string[], "Selected Device"=w333:string)
                n128 = Search 1D Array(1D array=w342, element=w333) -> (index of element=w331:i32)  [unwired: 1 in]
                n129 = Bundle By Name(cluster=T3 {"Up"=FALSE, "FUp"=FALSE, "Dn"=FALSE, "FDn"=FALSE, "Running?"=FALSE} ("element"), "Dn"=w334, "Running?"=w334) -> (w332:T3)
                n130 = Index Array(array=w341, index=w331) -> (element=w340:string)
                n131 = Replace Array Subset(array=w335, new element=w332, index=w331) -> (w336:T10)
                n132 = Bundle By Name(cluster=w337, "M"=w336) -> (w338:T4)
                n133 = case shown="True" w334 {
                  tunnel: w343 -> [w357 w363]
                  tunnel: [w355 w362] -> w339
                  tunnel: w340 -> [w356 w361]
                  tunnel: [250 ("f") 250 ("f")] -> w329
                  frame True {
                    n134 = call "Communication - Send Command Read.vi"("Fron?"=TRUE, "error in (no error)"=w357, "Action"=UDP_-_Command."Ramp Down", "Device IP Address"=w356) -> ("error out"=w355:errorcluster)  [unwired: 7 in]
                  }
                  frame False {
                    n135 = call "Communication - Send Command Read.vi"("Fron?"=TRUE, "error in (no error)"=w363, "Action"=UDP_-_Command."Stop", "Device IP Address"=w361) -> ("error out"=w362:errorcluster)  [unwired: 7 in]
                  }
                }
              }
              event "Fast down": Value Change {
                n136 = event-data() -> ("NewVal"=w373:bool)  [unwired: 1 in]
                n137 = Array Subset(array=w387, index=5) -> (w389:refnum<vi>[])  [unwired: 1 in]
                n138 = Select(t=w386, s=w373, f=w385) -> (s? t:f=w383:T1)
                n139 = for {
                  shift-right: [w405] -> w382
                  shift-left: w384 -> [w406]
                  tunnel: w389 -> [w404] mode=indexing
                  tunnel: w383 -> [w403]
                  n140 = property class="Bool"(reference=w404, error in=w406, "DisabledEnum"=w403) -> (error out=w405:errorcluster)  [unwired: 1 out]
                }
                n141 = Unbundle By Name(w376) -> ("M"=w374:T10, "Device IP"=w380:string[], "Device Name"=w381:string[], "Selected Device"=w372:string)
                n142 = Search 1D Array(1D array=w381, element=w372) -> (index of element=w370:i32)  [unwired: 1 in]
                n143 = Bundle By Name(cluster=T3 {"Up"=FALSE, "FUp"=FALSE, "Dn"=FALSE, "FDn"=FALSE, "Running?"=FALSE} ("element"), "FDn"=w373, "Running?"=w373) -> (w371:T3)
                n144 = Index Array(array=w380, index=w370) -> (element=w379:string)
                n145 = Replace Array Subset(array=w374, new element=w371, index=w370) -> (w375:T10)
                n146 = Bundle By Name(cluster=w376, "M"=w375) -> (w377:T4)
                n147 = case shown="True" w373 {
                  tunnel: w382 -> [w396 w402]
                  tunnel: [w395 w401] -> w378
                  tunnel: w379 -> [w394 w400]
                  tunnel: [250 ("f") 250 ("f")] -> w368
                  frame True {
                    n148 = call "Communication - Send Command Read.vi"("Fron?"=TRUE, "error in (no error)"=w396, "Action"=UDP_-_Command."Jog Down", "Device IP Address"=w394) -> ("error out"=w395:errorcluster)  [unwired: 7 in]
                  }
                  frame False {
                    n149 = call "Communication - Send Command Read.vi"("Fron?"=TRUE, "error in (no error)"=w402, "Action"=UDP_-_Command."Stop", "Device IP Address"=w400) -> ("error out"=w401:errorcluster)  [unwired: 7 in]
                  }
                }
              }
              event "MStop", "Stop Ch1", "Stop Ch2": Value Change {
                n150 = event-data() -> ()  [unwired: 1 in, 1 out]
                n151 = for {
                  shift-right: [w432] -> w427
                  shift-left: w428 -> [w433]
                  tunnel: w414 -> [w431] mode=indexing
                  tunnel: w415 -> [w430]
                  n152 = property class="Bool"(reference=w431, error in=w433, "DisabledEnum"=w430) -> (error out=w432:errorcluster)  [unwired: 1 out]
                }
                n153 = Unbundle By Name(w421) -> ("M"=w419:T10, "Device IP"=w425:string[], "Device Name"=w426:string[], "Selected Device"=w418:string)
                n154 = local write "Fast Up"(FALSE ("Fast Up")) -> ()
                n155 = local write "Fast down"(FALSE ("Fast down")) -> ()
                n156 = local write "Up"(FALSE ("Up")) -> ()
                n157 = local write "Down"(FALSE ("Down")) -> ()
                n158 = Search 1D Array(1D array=w426, element=w418) -> (index of element=w417:i32)  [unwired: 1 in]
                n159 = Index Array(array=w425, index=w417) -> (element=w424:string)
                n160 = Replace Array Subset(array=w419, new element=T3 {"Up"=FALSE, "FUp"=FALSE, "Dn"=FALSE, "FDn"=FALSE, "Running?"=FALSE} ("element"), index=w417) -> (w420:T10)
                n161 = Bundle By Name(cluster=w421, "M"=w420) -> (w422:T4)
                n162 = call "Communication - Send Command Read.vi"("Fron?"=TRUE, "error in (no error)"=w427, "Action"=UDP_-_Command."Stop", "Device IP Address"=w424) -> ("error out"=w423:errorcluster)  [unwired: 7 in]
              }
              event "Setpoint Ch1": Value Change {
                n163 = event-data() -> ("NewVal"=w440:sgl)  [unwired: 1 in]
                n164 = Unbundle By Name(w446) -> ("Device IP"=w447:string[], "Device Name"=w449:string[], "Selected Device"=w448:string)
                n165 = global read "Global - Test.vi" "Test"() -> (w443:T11)
                n166 = Search 1D Array(1D array=w449, element=w448) -> (index of element=w444:i32)  [unwired: 1 in]
                n167 = Index Array(array=w447, index=w444) -> (element=w436:string)
                n168 = Index Array(array=w443, index=w444) -> (element=w442:T12)
                n169 = Bundle By Name(cluster=w442, "Target Load"=w440) -> (w441:T12)
                n170 = Bundle By Name(cluster=T7 {"Test"={"Target Load"=0.0, "Target Disp"=0.0, "Rate"=0.0, "Speed"=0.0}, "Sensor"={"Name"=[], "Unit"=[], "Decimal Point"=[], "Ch Log"=[], "H Alarm"=[], "L Alarm"=[], "H Limit"=[], "L Limit"=[], "Filter"=[], "Gain"=[], "Calib Type"=[]}, "PID"={"SP"=0.0, "PV"=0.0, "kP"=0.0, "kI"=0.0, "kD"=0.0, "FF"=0.0, "Err Band"=0.0, "Max"=0, "Min"=0, "Ts"=0, "Out"=0, "Mode"=0}, "ADC"={"Active Ch"=[], "Filter Type"=0, "Post Filter"=[], "Gain"=[], "FS"=0, "IntOC"=0, "IntFC"=0, "SysOC"=0, "Cofficient"=[], "K"=[], "Max"=0}, "System"={"Out Type"=0, "Inverse"=0, "Monitor"=0, "Reserve"=0, "ACC Time"=0, "Pulse Rev"=0, "Stroke"=0, "Auto Off"=0, "Gear Ratio"=0.0, "Pitch"=0.0, "Max Speed"=0, "Jog Speed"=0, "Disp Coff"=0.0, "Max Load"=0}, "Index"=enum."Ch1", "Datalog"=enum."Ch1-Ch16"} ("Data"), "Test"=w441) -> (w439:T7)
                n171 = call "Communication - Send Command Read.vi"("Fron?"=TRUE, "error in (no error)"=w450, "Data"=w439, "Action"=UDP_-_Command."Write Test", "Device IP Address"=w436) -> ("error out"=w435:errorcluster)  [unwired: 6 in]
                n172 = call "Communication - Send Command Read.vi"("Fron?"=TRUE, "error in (no error)"=w435, "Action"=UDP_-_Command."Read Test", "Device IP Address"=w436) -> ("error out"=w434:errorcluster)  [unwired: 7 in]
              }
              event "Setpoint Rate": Value Change {
                n173 = event-data() -> ("NewVal"=w461:sgl)  [unwired: 1 in]
                n174 = Unbundle By Name(w467) -> ("Device IP"=w468:string[], "Device Name"=w470:string[], "Selected Device"=w469:string)
                n175 = global read "Global - Test.vi" "Test"() -> (w464:T11)
                n176 = Search 1D Array(1D array=w470, element=w469) -> (index of element=w465:i32)  [unwired: 1 in]
                n177 = Index Array(array=w468, index=w465) -> (element=w457:string)
                n178 = Index Array(array=w464, index=w465) -> (element=w463:T12)
                n179 = Bundle By Name(cluster=w463, "Rate"=w461) -> (w462:T12)
                n180 = Bundle By Name(cluster=T7 {"Test"={"Target Load"=0.0, "Target Disp"=0.0, "Rate"=0.0, "Speed"=0.0}, "Sensor"={"Name"=[], "Unit"=[], "Decimal Point"=[], "Ch Log"=[], "H Alarm"=[], "L Alarm"=[], "H Limit"=[], "L Limit"=[], "Filter"=[], "Gain"=[], "Calib Type"=[]}, "PID"={"SP"=0.0, "PV"=0.0, "kP"=0.0, "kI"=0.0, "kD"=0.0, "FF"=0.0, "Err Band"=0.0, "Max"=0, "Min"=0, "Ts"=0, "Out"=0, "Mode"=0}, "ADC"={"Active Ch"=[], "Filter Type"=0, "Post Filter"=[], "Gain"=[], "FS"=0, "IntOC"=0, "IntFC"=0, "SysOC"=0, "Cofficient"=[], "K"=[], "Max"=0}, "System"={"Out Type"=0, "Inverse"=0, "Monitor"=0, "Reserve"=0, "ACC Time"=0, "Pulse Rev"=0, "Stroke"=0, "Auto Off"=0, "Gear Ratio"=0.0, "Pitch"=0.0, "Max Speed"=0, "Jog Speed"=0, "Disp Coff"=0.0, "Max Load"=0}, "Index"=enum."Ch1", "Datalog"=enum."Ch1-Ch16"} ("Data"), "Test"=w462) -> (w460:T7)
                n181 = call "Communication - Send Command Read.vi"("Fron?"=TRUE, "error in (no error)"=w471, "Data"=w460, "Action"=UDP_-_Command."Write Test", "Device IP Address"=w457) -> ("error out"=w456:errorcluster)  [unwired: 6 in]
                n182 = call "Communication - Send Command Read.vi"("Fron?"=TRUE, "error in (no error)"=w456, "Action"=UDP_-_Command."Read Test", "Device IP Address"=w457) -> ("error out"=w455:errorcluster)  [unwired: 7 in]
              }
              event "Setpoint Ch2": Value Change {
                n183 = event-data() -> ("NewVal"=w482:sgl)  [unwired: 1 in]
                n184 = Unbundle By Name(w488) -> ("Device IP"=w489:string[], "Device Name"=w491:string[], "Selected Device"=w490:string)
                n185 = global read "Global - Test.vi" "Test"() -> (w485:T11)
                n186 = Search 1D Array(1D array=w491, element=w490) -> (index of element=w486:i32)  [unwired: 1 in]
                n187 = Index Array(array=w489, index=w486) -> (element=w478:string)
                n188 = Index Array(array=w485, index=w486) -> (element=w484:T12)
                n189 = Bundle By Name(cluster=w484, "Target Disp"=w482) -> (w483:T12)
                n190 = Bundle By Name(cluster=T7 {"Test"={"Target Load"=0.0, "Target Disp"=0.0, "Rate"=0.0, "Speed"=0.0}, "Sensor"={"Name"=[], "Unit"=[], "Decimal Point"=[], "Ch Log"=[], "H Alarm"=[], "L Alarm"=[], "H Limit"=[], "L Limit"=[], "Filter"=[], "Gain"=[], "Calib Type"=[]}, "PID"={"SP"=0.0, "PV"=0.0, "kP"=0.0, "kI"=0.0, "kD"=0.0, "FF"=0.0, "Err Band"=0.0, "Max"=0, "Min"=0, "Ts"=0, "Out"=0, "Mode"=0}, "ADC"={"Active Ch"=[], "Filter Type"=0, "Post Filter"=[], "Gain"=[], "FS"=0, "IntOC"=0, "IntFC"=0, "SysOC"=0, "Cofficient"=[], "K"=[], "Max"=0}, "System"={"Out Type"=0, "Inverse"=0, "Monitor"=0, "Reserve"=0, "ACC Time"=0, "Pulse Rev"=0, "Stroke"=0, "Auto Off"=0, "Gear Ratio"=0.0, "Pitch"=0.0, "Max Speed"=0, "Jog Speed"=0, "Disp Coff"=0.0, "Max Load"=0}, "Index"=enum."Ch1", "Datalog"=enum."Ch1-Ch16"} ("Data"), "Test"=w483) -> (w481:T7)
                n191 = call "Communication - Send Command Read.vi"("Fron?"=TRUE, "error in (no error)"=w492, "Data"=w481, "Action"=UDP_-_Command."Write Test", "Device IP Address"=w478) -> ("error out"=w477:errorcluster)  [unwired: 6 in]
                n192 = call "Communication - Send Command Read.vi"("Fron?"=TRUE, "error in (no error)"=w477, "Action"=UDP_-_Command."Read Test", "Device IP Address"=w478) -> ("error out"=w476:errorcluster)  [unwired: 7 in]
              }
              event "Speed": Value Change {
                n193 = event-data() -> ("NewVal"=w503:sgl)  [unwired: 1 in]
                n194 = Unbundle By Name(w509) -> ("Device IP"=w510:string[], "Device Name"=w512:string[], "Selected Device"=w511:string)
                n195 = global read "Global - Test.vi" "Test"() -> (w506:T11)
                n196 = Search 1D Array(1D array=w512, element=w511) -> (index of element=w507:i32)  [unwired: 1 in]
                n197 = Index Array(array=w510, index=w507) -> (element=w499:string)
                n198 = Index Array(array=w506, index=w507) -> (element=w505:T12)
                n199 = Bundle By Name(cluster=w505, "Speed"=w503) -> (w504:T12)
                n200 = Bundle By Name(cluster=T7 {"Test"={"Target Load"=0.0, "Target Disp"=0.0, "Rate"=0.0, "Speed"=0.0}, "Sensor"={"Name"=[], "Unit"=[], "Decimal Point"=[], "Ch Log"=[], "H Alarm"=[], "L Alarm"=[], "H Limit"=[], "L Limit"=[], "Filter"=[], "Gain"=[], "Calib Type"=[]}, "PID"={"SP"=0.0, "PV"=0.0, "kP"=0.0, "kI"=0.0, "kD"=0.0, "FF"=0.0, "Err Band"=0.0, "Max"=0, "Min"=0, "Ts"=0, "Out"=0, "Mode"=0}, "ADC"={"Active Ch"=[], "Filter Type"=0, "Post Filter"=[], "Gain"=[], "FS"=0, "IntOC"=0, "IntFC"=0, "SysOC"=0, "Cofficient"=[], "K"=[], "Max"=0}, "System"={"Out Type"=0, "Inverse"=0, "Monitor"=0, "Reserve"=0, "ACC Time"=0, "Pulse Rev"=0, "Stroke"=0, "Auto Off"=0, "Gear Ratio"=0.0, "Pitch"=0.0, "Max Speed"=0, "Jog Speed"=0, "Disp Coff"=0.0, "Max Load"=0}, "Index"=enum."Ch1", "Datalog"=enum."Ch1-Ch16"} ("Data"), "Test"=w504) -> (w502:T7)
                n201 = call "Communication - Send Command Read.vi"("Fron?"=TRUE, "error in (no error)"=w513, "Data"=w502, "Action"=UDP_-_Command."Write Test", "Device IP Address"=w499) -> ("error out"=w498:errorcluster)  [unwired: 6 in]
                n202 = call "Communication - Send Command Read.vi"("Fron?"=TRUE, "error in (no error)"=w498, "Action"=UDP_-_Command."Read Test", "Device IP Address"=w499) -> ("error out"=w497:errorcluster)  [unwired: 7 in]
              }
              event User Event {
                n203 = event-data() -> ()  [unwired: 1 in, 5 out]
                n204 = Unbundle By Name(w519) -> ("Device IP"=w518:string[])
                n205 = for {
                  shift-right: [w527] -> w521
                  shift-left: w520 -> [w528]
                  tunnel: w518 -> [w526] mode=indexing
                  n206 = call "Communication - Send Command Read.vi"("Fron?"=TRUE, "error in (no error)"=w528, "Action"=UDP_-_Command."Stop", "Device IP Address"=w526) -> ("error out"=w527:errorcluster)  [unwired: 7 in]
                }
              }
              event Panel Close? {
                n207 = event-data() -> ()  [unwired: 1 in, 4 out]
                n208 = Unbundle By Name(w539) -> ("Device Name"=w533:string[], "M"=w534:T10)
                n209 = for {
                  tunnel: w534 -> [w544] mode=indexing
                  tunnel: w538 -> [w543]
                  tunnel: [w543] -> w532
                  tunnel: w533 -> [w542] mode=indexing
                  tunnel: [w542] -> w531 mode=indexing if=w541
                  n210 = Unbundle By Name(w544) -> ("Running?"=w541:bool)
                }
                n211 = Empty Array?(array=w531) -> (empty?=w536:bool)
                n212 = case shown="True" w536 {
                  selector: w536 -> [w549 w559]
                  tunnel: [w554 w560] -> w537
                  tunnel: w532 -> [w546 w560]
                  tunnel: [w548 w558] -> w535
                  tunnel: w531 -> [w547 _]
                  tunnel: [w545 -1 ("f")] -> w530
                  tunnel: w529 -> [w545 _]
                  frame False {
                    n213 = Array To Spreadsheet String(delimiter (Tab)=", ", array=w547, 3:"" ("format string")) -> (spreadsheet string=w552:string)
                    n214 = Not(x=w549) -> (.not. x?=w548:bool)
                    n215 = call <vilib>:"Trim Whitespace.vi"("string"=w552) -> ("trimmed string"=w550:string)  [unwired: 1 in]
                    n216 = Format Into String(format string="%s still running.\nPlease stop the motor manually before leaving this page.", error in=w546, w550) -> (resulting string=w551:string, error out=w554:errorcluster)  [unwired: 1 in]
                    n217 = One Button Dialog(message=w551) -> ()  [unwired: 1 in, 1 out]
                  }
                  frame True {
                    n218 = Not(x=w559) -> (.not. x?=w558:bool)
                  }
                }
                n219 = event-data("Discard?"=w535) -> ()  [unwired: 1 in, 1 out]
              }
            }
          }
          frame "Read Data" {
            # "wy02 25: (kN)"
            n220 = Unbundle By Name(w593) -> ("Selected Device"=w592:string)
            n221 = global read "Global - Device.vi" "Device"() -> (w588:string[])
            n222 = global read "Global - System.vi" "System"() -> (w570:T13)
            n223 = Search 1D Array(1D array=w588, element=w592) -> (index of element=w568:i32)  [unwired: 1 in]
            n224 = global read "Global - Channel.vi" "Data"() -> (w589:T16)
            n225 = Index Array(array=w589, index=w568) -> (element=w590:T17)
            n226 = Index Array(array=w570, index=w568) -> (element=w569:T18)
            n227 = Unbundle By Name(w590) -> ("Channels.Ch1"=→"Data Ch1":sgl, "Channels.Ch2"=w562:sgl, "Channels.Ch3"=→"Data Ch3":sgl, "Channels.Ch4"=→"Data Ch4":sgl, "Event"=→"Event":T14, "Status"=→"Status":T15)
            "Data Ch2" <- w562
            n228 = Unbundle By Name(w569) -> ("Stroke"=w565:u32)
            n229 = Absolute Value(x=w562) -> (abs(x)=→"Slide":sgl)
            n230 = global read "Global - Unit.vi" "Unit"() -> (w584:T19)
            n231 = property on="Slide" class="Slide (strict)"(error in=w566, "Scale.Maximum"=w565, "Scale.Minimum"=0.0 ("Scale.Range:Minimum"), "Scale.Increment"=1.0 ("Scale.Range:Increment")) -> (error out=w567:errorcluster)  [unwired: 1 in, 1 out]
            n232 = Index Array(array=w584) -> (element=w585:T20)  [unwired: 1 in]
            n233 = Unbundle By Name(w585) -> ("Decimal Point"=w582:u8[], "Name"=w574:string[], "Unit"=w573:string[])
            n234 = Index Array(array=w582) -> (element #1=w581:u8, element #2=w580:u8, element #3=w576:u8, element #4=w575:u8)  [unwired: 4 in]
            n235 = for {
              tunnel: w574 -> [w599] mode=indexing
              tunnel: w573 -> [w598] mode=indexing
              i -> [w602]
              n236 = Format Into String(format string="%s: (%s)", initial string="", w599, w598) -> (resulting string=w597:string)  [unwired: 1 in, 1 out]
              n237 = case shown="3" w602 {
                tunnel: w598 -> [w604 w606 _ _]
                tunnel: w597 -> [w603 w605 w607 w608]
                frame 0, Default {
                  "Unit Ch1" <- w604
                  "Unit Ch1b" <- w604
                  "Label Ch1" <- w603
                }
                frame 1 {
                  "Unit Ch2" <- w606
                  "Unit Ch2b" <- w606
                  "Label Ch2" <- w605
                }
                frame 2 {
                  "Label Ch3" <- w607
                }
                frame 3 {
                  "Label Ch4" <- w608
                }
              }
            }
            n238 = property on="Data Ch1" class="DigNum (strict)"(error in=w567, "Precision"=w581) -> (error out=w583:errorcluster)  [unwired: 1 in, 1 out]
            n239 = property on="Data Ch2" class="DigNum (strict)"(error in=w583, "Precision"=w580) -> (error out=w579:errorcluster)  [unwired: 1 in, 1 out]
            n240 = property on="Data Ch3" class="DigNum (strict)"(error in=w579, "Precision"=w576) -> (error out=w578:errorcluster)  [unwired: 1 in, 1 out]
            n241 = property on="Data Ch4" class="DigNum (strict)"(error in=w578, "Precision"=w575) -> (error out=w577:errorcluster)  [unwired: 1 in, 1 out]
          }
          frame "Close" {
            n242 = control-ref of="This VI"() -> (w611:refnum<vi>)
            n243 = invoke class="VI" method="FP.Close"(reference=w611, error in=w609) -> (error out=w610:errorcluster)  [unwired: 1 in, 2 out]
          }
        }
      }
      frame Error {
        n244 = Unbundle By Name(w617) -> ("source"=w622:string)
        n245 = call <vilib>:"Clear Errors.vi"("error in (no error)"=w617) -> ("error out"=w619:errorcluster)  [unwired: 5 in, 1 out]
        n246 = Concatenate Strings("Manual Control" ("string"), " - " ("string"), w622) -> (w620:string)
        n247 = call "General - Error Log eFGV.vi"("eFGV States"=eFGV_States."Write", "error in (no error)"=w619, "Error In"=w620) -> ("error out"=w618:errorcluster)  [unwired: 6 in, 2 out]
        n248 = Wait (ms)(milliseconds to wait=u32 100) -> ()  [unwired: 1 out]
      }
    }
  }
